vi "CalculateRadius.vi"(2 "Scan Type":T1(ring), 3 "Points per Scan":u8, 4 "Spacing (V)":dbl) -> (0 "Maximum Voltage (V)":dbl, 1 "Radius (V)":dbl)   [LabVIEW 2011]
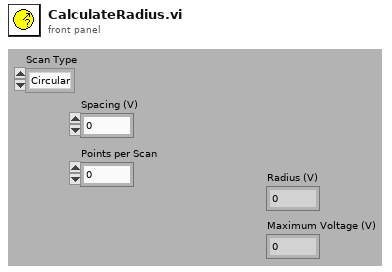
[diagram p1: front panel]
types:
  T1 = enum8{"Circular", "Square", "Hexagonal", "FilledSquare"}
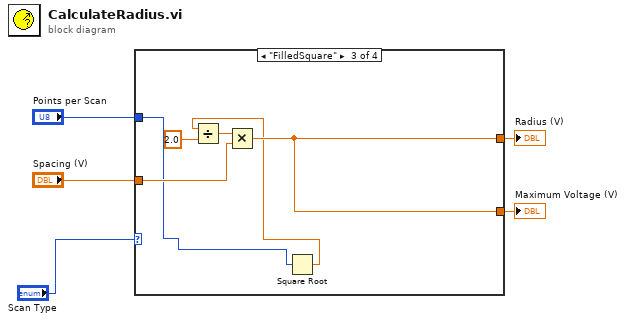
[diagram p0: block diagram]
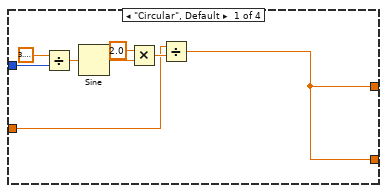
[diagram p2: hidden frame]
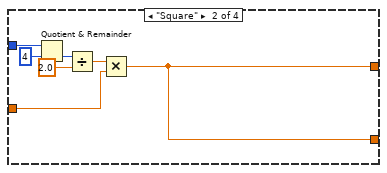
[diagram p3: hidden frame]
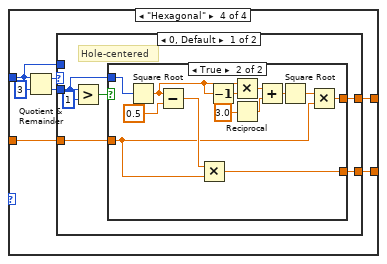
[diagram p4: hidden frame]
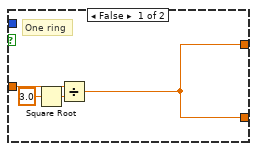
[diagram p5: hidden frame]
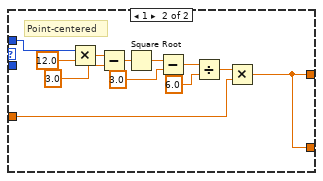
[diagram p6: hidden frame]
diagram:
  n1 = case shown="\"FilledSquare\"" "Scan Type" {
    tunnel: "Points per Scan" -> [w9 w20 w22 w27]
    tunnel: "Spacing (V)" -> [w7 w15 w24 w30]
    tunnel: [w6 w14 w23 w29] -> w3
    tunnel: [w6 w14 w23 w28] -> w2
    frame "Circular", Default {
      n2 = Divide(x=3.141592653589793, y=w9) -> (x/y=w12:dbl)
      n3 = Sine(x=w12) -> (sin(x)=w11:dbl)
      n4 = Multiply(x=2.0, y=w11) -> (x*y=w8:dbl)
      n5 = Divide(x=w7, y=w8) -> (x/y=w6:dbl)
    }
    frame "Square" {
      n6 = Quotient & Remainder(x=w20, y=u8 4) -> (floor(x/y)=w18:u8)  [unwired: 1 out]
      n7 = Divide(x=w18, y=2.0) -> (x/y=w16:dbl)
      n8 = Multiply(x=w16, y=w15) -> (x*y=w14:dbl)
    }
    frame "FilledSquare" {
      n9 = Square Root(x=w22) -> (sqrt(x)=w21:dbl)
      n10 = Divide(x=w21, y=2.0) -> (x/y=w25:dbl)
      n11 = Multiply(x=w25, y=w24) -> (x*y=w23:dbl)
    }
    frame "Hexagonal" {
      n12 = Quotient & Remainder(x=w27, y=u8 3) -> (x-y*floor(x/y)=w32:u8, floor(x/y)=w31:u8)
      n13 = case shown="0, Default" w32 {
        tunnel: w31 -> [w34 _]
        tunnel: w30 -> [w37 w58]
        tunnel: [w36 w57] -> w29
        tunnel: [w35 w57] -> w28
        tunnel: w27 -> [_ w68]
        frame 0, Default {
          # "Hole-centered"
          n14 = Greater?(x=w34, y=u8 1) -> (0:w38:bool)
          n15 = case shown="True" w38 {
            tunnel: w37 -> [w43 w44]
            tunnel: [w40 w45] -> w36
            tunnel: [w40 w54] -> w35
            tunnel: w34 -> [_ w56]
            frame False {
              # "One ring"
              n16 = Square Root(x=3.0) -> (sqrt(x)=w42:dbl)
              n17 = Divide(x=w43, y=w42) -> (x/y=w40:dbl)
            }
            frame True {
              n18 = Square Root(x=w56) -> (sqrt(x)=w51:dbl)
              n19 = Subtract(x=w51, y=0.5) -> (x-y=w53:dbl)
              n20 = Multiply(x=w53, y=w44) -> (x*y=w54:dbl)
              n21 = Decrement(x=w51) -> (x-1=w52:dbl)
              n22 = Multiply(x=w51, y=w52) -> (x*y=w50:dbl)
              n23 = Reciprocal(x=3.0) -> (1/x=w49:dbl)
              n24 = Add(x=w50, y=w49) -> (x+y=w47:dbl)
              n25 = Square Root(x=w47) -> (sqrt(x)=w46:dbl)
              n26 = Multiply(x=w46, y=w44) -> (x*y=w45:dbl)
            }
          }
        }
        frame 1 {
          # "Point-centered"
          n27 = Multiply(x=w68, y=12.0) -> (x*y=w66:dbl)
          n28 = Subtract(x=w66, y=3.0) -> (x-y=w64:dbl)
          n29 = Square Root(x=w64) -> (sqrt(x)=w63:dbl)
          n30 = Subtract(x=w63, y=3.0) -> (x-y=w61:dbl)
          n31 = Divide(x=w61, y=6.0) -> (x/y=w59:dbl)
          n32 = Multiply(x=w59, y=w58) -> (x*y=w57:dbl)
        }
      }
    }
  }
  "Radius (V)" <- w3
  "Maximum Voltage (V)" <- w2
